vi "Pre Launch Init.vi"(11 "Nested in":refnum<class "Network Test.lvclass">) -> (0 "error out":errorcluster, 3 "Nested out":refnum<class "Network Test.lvclass">)   [LabVIEW 2017, in "Network Test.lvlib" / "Network Test.lvclass"]
doc: "(<B>Filename</B>: Actor Framework.lvlib:Actor.lvclass:Pre Launch Init.vi)\n\nDefines behavior that occurs after the Launch Nested Actor method is invoked but before the actor's Actor Core method begins running.\n\nBy default, this method does nothing. A descendant class may override it to define behavior."
uses:
  Network Test.lvclass
  Ping Test Configuration.ctl
  Network Test.lvclass/Network Test.ctl
  Test/Test/Test.lvclass
  Network Test.lvlib
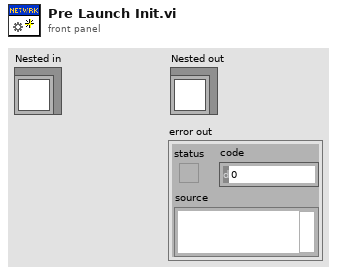
[diagram p1: front panel]
types:
  T1 = typedef "Network Test.lvlib/Ping Test Configuration.ctl" = cluster{"IP/Address":string, "PacketSize":i32, "timeout":i32, "Packet Count":i32, "Min Expected Packed Return %":dbl, "Ping Result":cluster{"Result?":bool, "Actual Packet Return %":dbl}}
  T2 = cluster{"Result?":bool, "Actual Packet Return %":dbl}
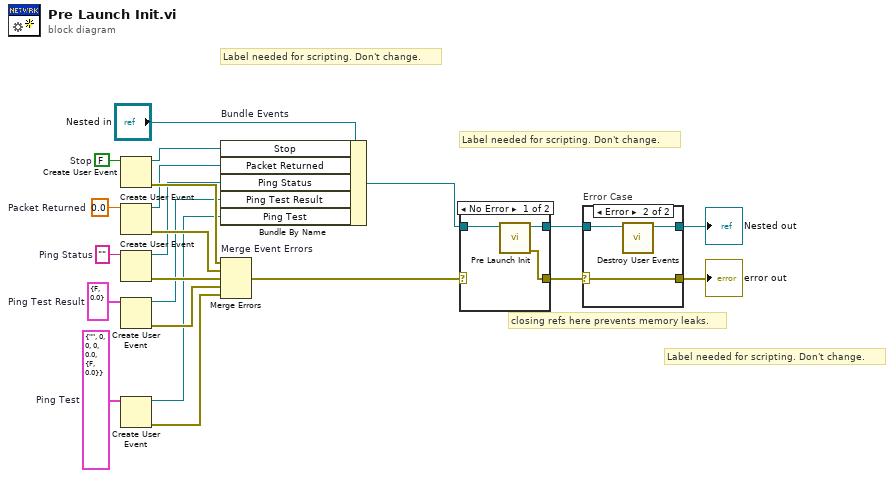
[diagram p0: block diagram]
diagram:
  w3 = T1 {"IP/Address"="", "PacketSize"=0, "timeout"=0, "Packet Count"=0, "Min Expected Packed Return %"=0.0, "Ping Result"={"Result?"=FALSE, "Actual Packet Return %"=0.0}}  # Ping Test
  w6 = T2 {"Result?"=FALSE, "Actual Packet Return %"=0.0}  # Ping Test Result
  w9 = ""  # Ping Status
  w12 = 0.0  # Packet Returned
  w21 = FALSE  # Stop
  # "Label needed for scripting. Don't change."
  # "Label needed for scripting. Don't change."
  # "Label needed for scripting. Don't change."
  # "closing refs here prevents memory leaks."
  n1 = Create User Event(user event datatype=w21) -> (user event=w18:refnum<user-event>, error out=w20:errorcluster)  [unwired: 1 in]
  n2 = Create User Event(user event datatype=w12) -> (user event=w11:refnum<user-event>, error out=w10:errorcluster)  [unwired: 1 in]
  n3 = Create User Event(user event datatype=w9) -> (user event=w8:refnum<user-event>, error out=w7:errorcluster)  [unwired: 1 in]
  n4 = Create User Event(user event datatype=w6) -> (user event=w5:refnum<user-event>, error out=w4:errorcluster)  [unwired: 1 in]
  n5 = Create User Event(user event datatype=w3) -> (user event=w2:refnum<user-event>, error out=w1:errorcluster)  [unwired: 1 in]
  n6 = Bundle By Name "Bundle Events"(cluster="Nested in", "Stop"=w18, "Packet Returned"=w11, "Ping Status"=w8, "Ping Test Result"=w5, "Ping Test"=w2) -> (w15:refnum<class "Network Test.lvclass">)
  n7 = Merge Errors "Merge Event Errors"(w20, w10, w7, w4, w1) -> (w14:errorcluster)
  n8 = case shown="No Error" w14 {
    selector: w14 -> [_ w27]
    tunnel: [w25 w26] -> w16
    tunnel: w15 -> [w24 w26]
    tunnel: [w23 w27] -> w13
    frame No Error {
      n9 = call-parent "Pre Launch Init.vi"("Actor in"=w24) -> ("error out"=w23:errorcluster, "Actor out"=w25:refnum<class "Network Test.lvclass">)  [unwired: 9 in]
    }
    frame Error {
    }
  }
  n10 = case "Error Case" shown="Error" w13 {
    selector: w13 -> [w28 w32]
    tunnel: w16 -> [w29 w31]
    tunnel: [w29 w30] -> w19
    tunnel: [w28 w32] -> w17
    frame No Error {
    }
    frame Error {
      n11 = call "Destroy User Events.vi"("UI Template in"=w31) -> ("UI Template out"=w30:refnum<class "Network Test.lvclass">)  [unwired: 10 in]
    }
  }
  "error out" <- w17
  "Nested out" <- w19
